vi "DataLog Build Log Path.vi"(5 "database path":path, 7 "tag":string, 11 "error in (no error)":errorcluster) -> (4 "tag log directory":path, 15 "error out":errorcluster)   [LabVIEW 2012]
doc: "Return the tag's log directory based on the database path and the tag's name."
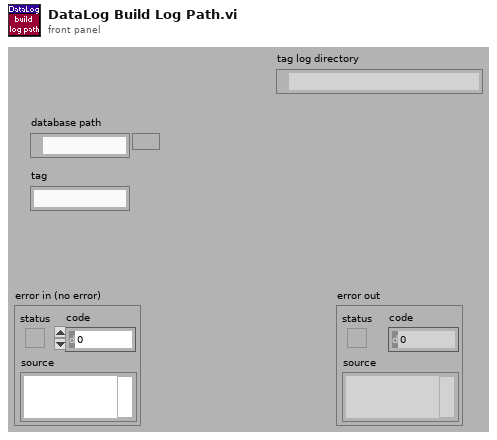
[diagram p1: front panel]
types:
  T1 = typedef "et_DataLog Meta Tag Specifier.ctl" = enum32{"warn_lo", "warn_hi", "A_lo", "A_hi", "B_lo", "B_hi", "C_lo", "C_hi", "D_lo", "D_hi", "E_lo", "E_hi", "F_lo", "F_hi", "G_lo", "G_hi", "H_lo", "H_hi", "I_lo", "I_hi", "J_lo", "J_hi", "K_lo", "K_hi", "L_lo", "L_hi", "M_lo", "M_hi", "N_lo", "N_hi", "min", "max", "not a meta"}
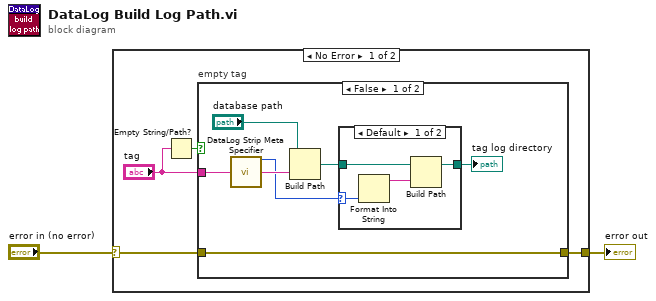
[diagram p0: block diagram]
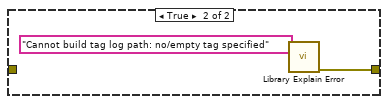
[diagram p3: hidden frame]
diagram:
  n1 = case shown="No Error" "error in (no error)" {
    selector: "error in (no error)" -> [w5 w21]
    tunnel: [w4 w21] -> w2
    frame No Error {
      n2 = Empty String/Path?(string/path="tag") -> (empty?=w6:bool)
      n3 = case "empty tag" shown="False" w6 {
        tunnel: "tag" -> [w8 _]
        tunnel: w5 -> [w7 _]
        tunnel: [w7 w20] -> w4
        frame False {
          n4 = call "DataLog Strip Meta Specifier.vi"("tag"=w8) -> ("meta specifier"=w12:T1, "base tag"=w13:string)  [unwired: 13 in]
          n5 = Build Path(base path="database path", name or relative path=w13) -> (appended path=w11:path)
          n6 = case shown="Default" w12 {
            selector: w12 -> [w15 _]
            tunnel: w11 -> [w17 w18]
            tunnel: [w16 w18] -> w10
            frame Default {
              n7 = Format Into String(w15) -> (resulting string=w14:string)  [unwired: 3 in, 1 out]
              n8 = Build Path(base path=w17, name or relative path=w14) -> (appended path=w16:path)
            }
            frame "not a meta" {
            }
          }
          "tag log directory" <- w10
        }
        frame True {
          n9 = call "Library Explain Error.vi"("explanation prefix (none)"="Cannot build tag log path: no/empty tag specified") -> ("explained error"=w20:errorcluster)  [unwired: 14 in]
        }
      }
    }
    frame Error {
    }
  }
  "error out" <- w2
